vi "PostProcess.vi"(8 "error in (no error)":errorcluster, 10 "Variant in":variant, 11 "ONNX YOLO Class in":refnum<class "ONNX YOLO Class.lvclass">) -> (0 "error out":errorcluster, 2 "Variant out":variant, 3 "ONNX YOLO Class out":refnum<class "ONNX YOLO Class.lvclass">)   [LabVIEW 2017, in "ONNX YOLO Class Library.lvlib" / "ONNX YOLO Class.lvclass"]
uses:
  ONNX YOLO Class.lvclass
  <vilib>/picture/picture.llb/imagedata.ctl
  TypeDef/Circle.ctl
  ONNX YOLO Class Library.lvlib
panel:
  out "Circles":T1[](array[typedef])
  out "image out":picture
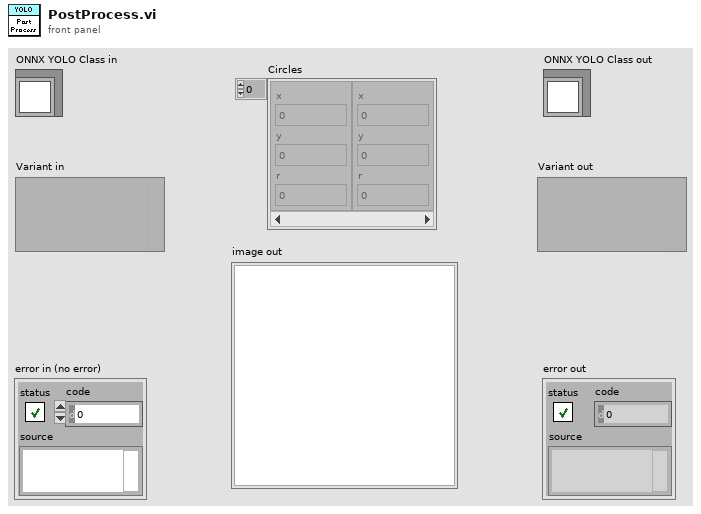
[diagram p1: front panel]
types:
  T1 = typedef "ONNX YOLO Class Library.lvlib/Circle.ctl" = cluster{"x":sgl, "y":sgl, "r":sgl}
  T2 = typedef "imagedata.ctl" = cluster{"image type":i32, "image depth":i32, "image":u8[], "mask":u8[], "colors":u32[], "Rectangle":cluster{"left":i16, "top":i16, "right":i16, "bottom":i16}}
  T3 = typedef "ONNX Class Library.lvlib/Introspection.ctl" = cluster{"Count":i32, "Shapes":T4[]}
  T4 = typedef "ONNX Class Library.lvlib/IO.ctl" = cluster{"Name":string, "DimCount":i32, "Type Index":i32, "Type Name":string, "Dims":i64[]}
  T5 = typedef "ONNX YOLO Class Library.lvlib/Box.ctl" = cluster{"conf":sgl, "x_center":sgl, "y_center":sgl, "width":sgl, "height":sgl, "x1":sgl, "y1":sgl, "x2":sgl, "y2":sgl}
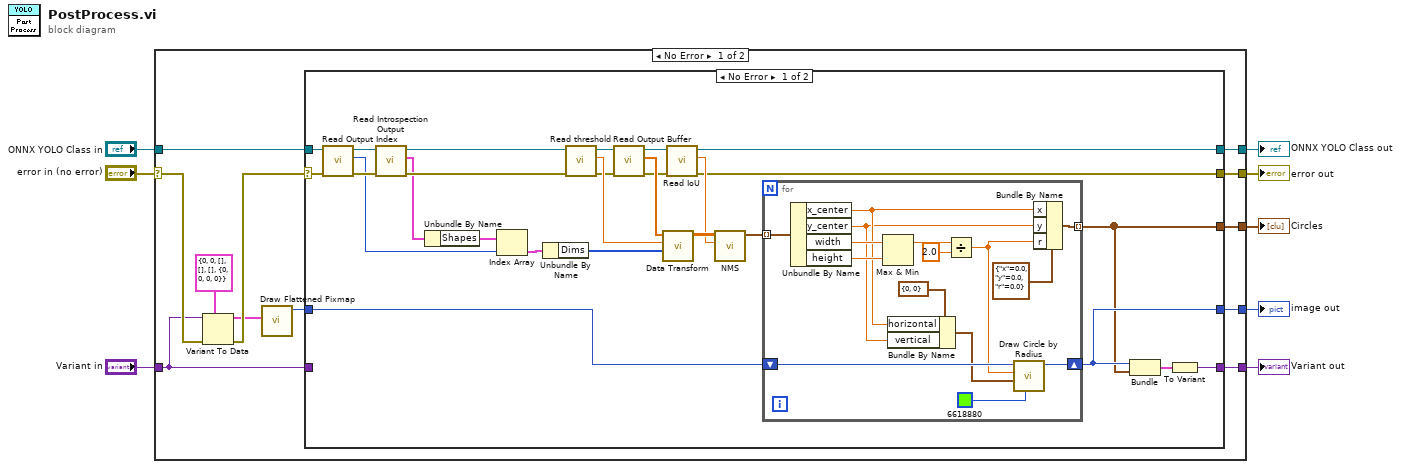
[diagram p0: block diagram]
diagram:
  n1 = case shown="No Error" "error in (no error)" {
    selector: "error in (no error)" -> [w19 w67]
    tunnel: "Variant in" -> [w14 w68]
    tunnel: "ONNX YOLO Class in" -> [w18 w69]
    tunnel: [w16 w69] -> w5
    tunnel: [w13 w68] -> w4
    tunnel: [w15 w67] -> w3
    tunnel: [w17 _] -> w2
    tunnel: [w9 _] -> w1
    frame No Error {
      n2 = Variant To Data(error in=w19, type=T2 {"image type"=0, "image depth"=0, "image"=[], "mask"=[], "colors"=[], "Rectangle"={"left"=0, "top"=0, "right"=0, "bottom"=0}} ("image data"), Variant=w14) -> (data=w11:T2, error out=w20:errorcluster)
      n3 = call <vilib>:"Draw Flattened Pixmap.vi"("image data"=w11) -> ("new picture"=w10:picture)  [unwired: 8 in]
      n4 = case shown="No Error" w20 {
        selector: w20 -> [w38 w65]
        tunnel: w18 -> [w39 w66]
        tunnel: [w24 w63] -> w17
        tunnel: [w25 w66] -> w16
        tunnel: [w26 w65] -> w15
        tunnel: w14 -> [_ w64]
        tunnel: [w21 w64] -> w13
        tunnel: w10 -> [w42 w63]
        tunnel: [w23 _] -> w9
        frame No Error {
          n5 = call-dynamic "Read Output Index.vi"("error in (no error)"=w38, "ONNX Class in"=w39) -> ("error out"=w35:errorcluster, "Output Index"=w32:i32, "ONNX Class out"=w37:refnum<class "ONNX YOLO Class.lvclass">)  [unwired: 7 in]
          n6 = call-dynamic "Read Introspection Output.vi"("error in (no error)"=w35, "ONNX Class in"=w37) -> ("error out"=w34:errorcluster, "Introspection"=w33:T3, "ONNX Class out"=w36:refnum<class "ONNX YOLO Class.lvclass">)  [unwired: 7 in]
          n7 = Unbundle By Name(w33) -> ("Shapes"=w41:T4[])
          n8 = Index Array(array=w41, index=w32) -> (element=w40:T4)
          n9 = Unbundle By Name(w40) -> ("Dims"=w31:i64[])
          n10 = call-dynamic "Read threshold.vi"("error in (no error)"=w34, "ONNX YOLO Class in"=w36) -> ("error out"=w29:errorcluster, "threshold"=w43:sgl, "ONNX YOLO Class out"=w30:refnum<class "ONNX YOLO Class.lvclass">)  [unwired: 7 in]
          n11 = call-dynamic "Read Output Buffer.vi"("error in (no error)"=w29, "ONNX Class in"=w30) -> ("error out"=w27:errorcluster, "Output Buffer"=w45:sgl[], "ONNX Class out"=w28:refnum<class "ONNX YOLO Class.lvclass">)  [unwired: 7 in]
          n12 = call "Data Transform.vi"("dim"=w31, "threshold"=w43, "Array in"=w45) -> ("Array out"=w47:sgl[][])  [unwired: 8 in]
          n13 = call-dynamic "Read IoU.vi"("error in (no error)"=w27, "ONNX YOLO Class in"=w28) -> ("error out"=w26:errorcluster, "IoU"=w44:sgl, "ONNX YOLO Class out"=w25:refnum<class "ONNX YOLO Class.lvclass">)  [unwired: 7 in]
          n14 = call "NMS.vi"("IoU"=w44, "Array in"=w47) -> ("Box out"=w46:T5[])  [unwired: 9 in]
          n15 = for {
            shift-right: [w61] -> w24
            shift-left: w42 -> [w62]
            tunnel: w46 -> [w57] mode=indexing
            tunnel: [w48] -> w23 mode=indexing
            n16 = Unbundle By Name(w57) -> ("x_center"=w51:sgl, "y_center"=w50:sgl, "width"=w56:sgl, "height"=w55:sgl)
            n17 = Max & Min(x=w56, y=w55) -> (max(x,y)=w54:sgl)  [unwired: 1 out]
            n18 = Bundle By Name(cluster=cluster{"horizontal":i16, "vertical":i16} {"horizontal"=0, "vertical"=0} ("pixel center"), "horizontal"=w51, "vertical"=w50) -> (w58:cluster{"horizontal":i16, "vertical":i16})
            n19 = Divide(x=w54, y=sgl 2.0) -> (x/y=w49:sgl)
            n20 = call <vilib>:"Draw Circle by Radius.vi"("color(black)"=u32 6618880, "pixel center"=w58, "radius"=w49, "picture"=w62) -> ("new picture"=w61:picture)  [unwired: 7 in]
            n21 = Bundle By Name(cluster=T1 {"x"=0.0, "y"=0.0, "r"=0.0} ("Circle"), "x"=w51, "y"=w50, "r"=w49) -> (w48:T1)
          }
          n22 = Bundle("new picture"=w24, w23) -> (w22:cluster{"new picture":picture, T1[]})  [unwired: 1 in]
          n23 = To Variant(anything=w22) -> (Variant=w21:variant)
        }
        frame Error {
        }
      }
    }
    frame Error {
    }
  }
  "error out" <- w3
  "ONNX YOLO Class out" <- w5
  "Variant out" <- w4
  "image out" <- w2
  "Circles" <- w1
